vi "generateCheckCode.vi"(1 "Data":string) -> (0 "CheckCode":string)   [LabVIEW 2010]
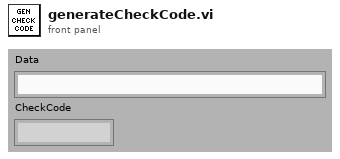
[diagram p1: front panel]
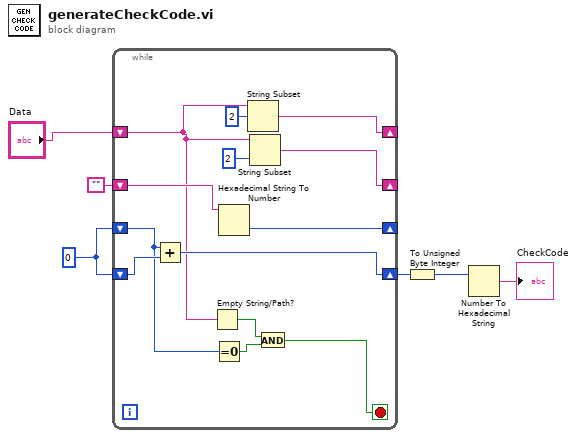
[diagram p0: block diagram]
diagram:
  w4 = u32 0
  n1 = while {
    shift-right: [w17] -> _
    shift-left: "Data" -> [w11]
    shift-right: [w16] -> _
    shift-left: "" ("String") -> [w15]
    shift-right: [w14] -> _
    shift-left: w4 -> [w10]
    shift-right: [w12] -> w2
    shift-left: w4 -> [w13]
    stop <- w7 stop-if-true
    n2 = Add(x=w10, y=w13) -> (x+y=w12:u32)
    n3 = Empty String/Path?(string/path=w11) -> (empty?=w8:bool)
    n4 = Equal To 0?(x=w10) -> (x = 0?=w9:bool)
    n5 = Hexadecimal String To Number(string=w15) -> (number=w14:u32)  [unwired: 2 in, 1 out]
    n6 = String Subset(string=w11, offset (0)=2) -> (substring=w17:string)  [unwired: 1 in]
    n7 = String Subset(string=w11, length (rest)=2 ("offset (0)")) -> (substring=w16:string)  [unwired: 1 in]
    n8 = And(x=w8, y=w9) -> (x .and. y?=w7:bool)
  }
  n9 = To Unsigned Byte Integer(number=w2) -> (unsigned 8bit integer=w1:u8)
  n10 = Number To Hexadecimal String(2:w1) -> (0:→"CheckCode":string)  [unwired: 1 in]
